vi "Pat message.vi"(8 "error in (no error)":errorcluster, 11 "Guardian in":refnum<class "Guardian.lvclass">) -> (0 "error out":errorcluster, 1 "Data":string[](array[string]), 2 "Message name":string, 3 "Guardian out":refnum<class "Guardian.lvclass">)   [LabVIEW 2026, in "TALOS.lvlib" / "Guardian.lvlib" / "Guardian.lvclass"]
uses:
  Guardian.lvclass
  C:/LabVIEW Code/TALOS/talos/Ancestor/Ancestor/Ancestor.lvclass
  Ancestor/Ancestor/Ancestor.lvclass/Ancestor.ctl
  Ancestor/Ancestor/Ancestor.lvclass
  TALOS.lvlib
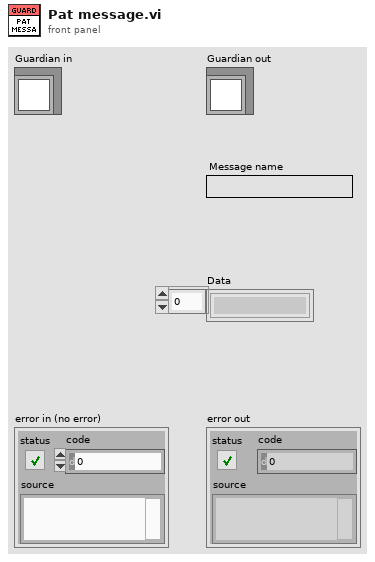
[diagram p1: front panel]
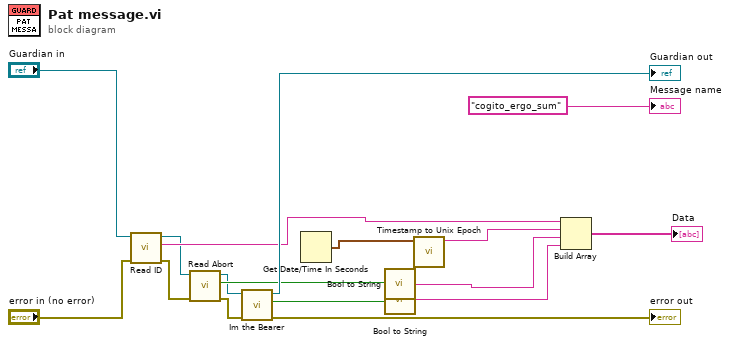
[diagram p0: block diagram]
diagram:
  n1 = call "Read ID.vi"("error in (no error)"="error in (no error)", "Ancestor in"="Guardian in") -> ("error out"=w8:errorcluster, "ID"=w15:string, "Ancestor out"=w9:refnum<class "Guardian.lvclass">)  [unwired: 7 in]
  n2 = call "Read Abort.vi"("error in (no error)"=w8, "Guardian in"=w9) -> ("error out"=w7:errorcluster, "Abort"=w10:bool, "Guardian out"=w6:refnum<class "Guardian.lvclass">)  [unwired: 7 in]
  n3 = call "Im the Bearer.vi"("error in (no error)"=w7, "Guardian in"=w6) -> ("error out"=→"error out":errorcluster, "I'm the Bearer"=w11:bool, "Guardian out"=→"Guardian out":refnum<class "Guardian.lvclass">)  [unwired: 7 in]
  n4 = Get Date/Time In Seconds() -> (seconds since 1Jan1904=w16:timestamp)
  n5 = call "Bool to String.vi"("Boolean"=w10) -> ("String"=w3:string)
  n6 = call "Bool to String.vi"("Boolean"=w11) -> ("String"=w2:string)
  n7 = call "Timestamp to Unix Epoch.vi"("seconds since 1Jan1904"=w16) -> ("String"=w4:string)  [unwired: 10 in]
  n8 = Build Array(w15, w4, w3, w2) -> (→"Data":string[])
  "Message name" <- "cogito_ergo_sum" ("Message")
